vi "serial.vi"() -> ()   [LabVIEW 2016]
uses:
  <vilib>/Instr/_visa.llb/VISA Configure Serial Port (Instr).vi
panel:
  out "Boolean array":bool[](array[boolean])
  in  "Array":bool[](array[boolean])
  in  "Stop Button":bool
  in  "Cluster":T1={"VISA resource name"="", "baud rate (9600)"=9600, "parity (0:none)"=enum."None", "stop bits (10: 1 bit)"=10, "flow control (0:none)"=0, "timeout (10sec)"=10000, "data bits (8)"=8} {"stop bits (10: 1 bit)" items=["1.0"=10, "1.5"=15, "2.0"=20]; "flow control (0:none)" items=["None", "XON/XOFF", "RTS/CTS", "XON/XOFF & RTS/CTS", "DTR/DSR", "XON/XOFF & DTR/DSR"]; "data bits (8)" min=5 max=8 step=1}
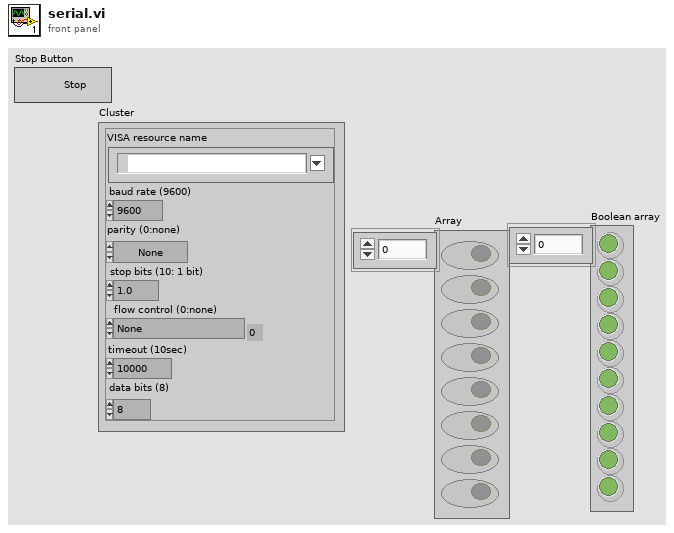
[diagram p1: front panel]
types:
  T1 = cluster{"VISA resource name":refnum<visa-resource-name>, "baud rate (9600)":u32, "parity (0:none)":enum16{"None", "Odd", "Even", "Mark", "Space"}, "stop bits (10: 1 bit)":u16, "flow control (0:none)":u16, "timeout (10sec)":u32, "data bits (8)":u16}
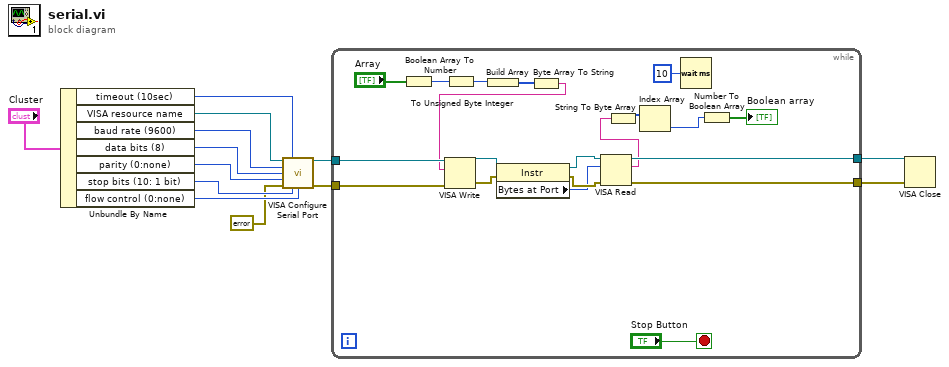
[diagram p0: block diagram]
diagram:
  n1 = Unbundle By Name("Cluster") -> ("timeout (10sec)"=w12:u32, "VISA resource name"=w11:refnum<visa-resource-name>, "baud rate (9600)"=w10:u32, "data bits (8)"=w9:u16, "parity (0:none)"=w8:enum16{"None", "Odd", "Even", "Mark", "Space"}, "stop bits (10: 1 bit)"=w7:u16, "flow control (0:none)"=w6:u16)
  n2 = call-poly "VISA Configure Serial Port"("VISA resource name"=w11, "timeout (10sec)"=w12, "baud rate (9600)"=w10, "data bits (8)"=w9, "parity (0:none)"=w8, "error in (no error)"=errorcluster {"status"=FALSE, "code"=0, "source"=""}, "stop bits (10: 1 bit)"=w7, "flow control (0:none)"=w6) -> ("VISA resource name out"=w5:refnum<visa-resource-name>, "error out"=w4:errorcluster)  [unwired: 6 in]
  n3 = while {
    tunnel: w5 -> [w32]
    tunnel: w4 -> [w33]
    tunnel: [w31] -> w2
    tunnel: [w30] -> w1
    stop <- "Stop Button" stop-if-true
    n4 = Boolean Array To Number(Boolean array="Array") -> (number=w21:u32)
    n5 = To Unsigned Byte Integer(number=w21) -> (unsigned 8bit integer=w20:u8)
    n6 = Build Array(w20) -> (w19:u8[])
    n7 = Byte Array To String(unsigned byte array=w19) -> (string=w18:string)
    n8 = VISA Write(VISA resource name=w32, write buffer=w18, error in (no error)=w33) -> (VISA resource name out=w27:refnum<visa-resource-name>, error out=w26:errorcluster)  [unwired: 1 out]
    n9 = property class="Instr"(reference=w27, error in=w26) -> (reference out=w25:refnum<visa-resource-name>, error out=w24:errorcluster, "Bytes at Port"=w23:u32)
    n10 = VISA Read(VISA resource name=w25, byte count=w23, error in (no error)=w24) -> (VISA resource name out=w31:refnum<visa-resource-name>, read buffer=w14:string, error out=w30:errorcluster)  [unwired: 1 out]
    n11 = String To Byte Array(string=w14) -> (unsigned byte array=w17:u8[])
    n12 = Index Array(array=w17) -> (element=w16:u8)  [unwired: 1 in]
    n13 = Wait (ms)(milliseconds to wait=u32 10) -> ()  [unwired: 1 out]
    n14 = Number To Boolean Array(number=w16) -> (Boolean array=→"Boolean array":bool[])
  }
  n15 = VISA Close(VISA resource name=w2, error in (no error)=w1) -> ()  [unwired: 1 out]
